vi "MakeReference.vi"(8 "error in (no error)":errorcluster, 10 "DatatoRef":T1, 11 "Refnum in":refnum<k34>) -> (0 "error out":errorcluster, 3 "Refnum out":refnum<k34>)   [LabVIEW 2021]
uses:
  Typedefs/DataToRef.ctl
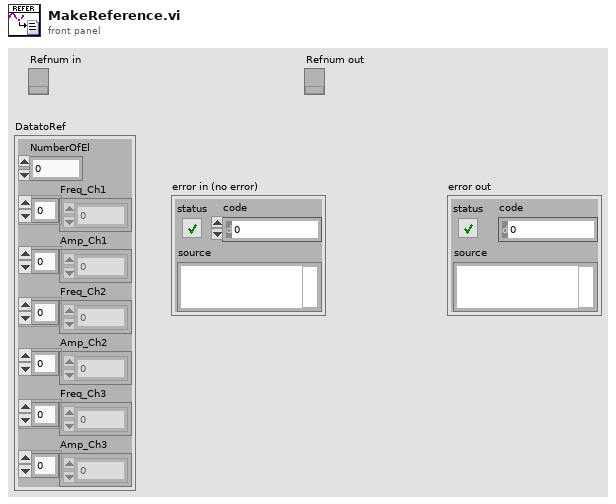
[diagram p1: front panel]
types:
  T1 = typedef "DataToRef.ctl" = cluster{"NumberOfEl":dbl, "Freq_Ch1":dbl[], "Amp_Ch1":dbl[], "Freq_Ch2":dbl[], "Amp_Ch2":dbl[], "Freq_Ch3":dbl[], "Amp_Ch3":dbl[]}
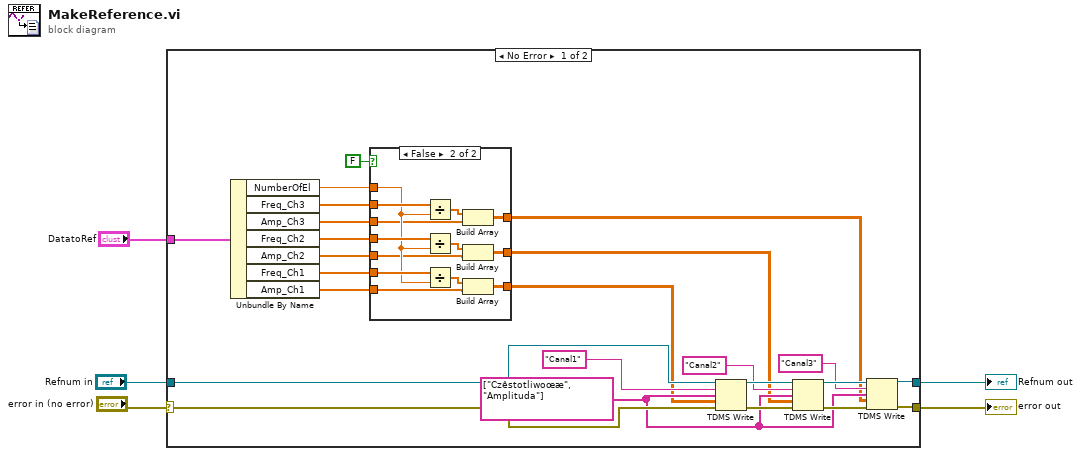
[diagram p0: block diagram]
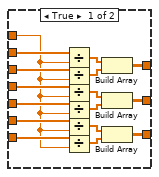
[diagram p2: hidden frame]
diagram:
  n1 = case shown="No Error" "error in (no error)" {
    selector: "error in (no error)" -> [w29 w59]
    tunnel: [w21 w59] -> w4
    tunnel: [w22 w60] -> w3
    tunnel: "Refnum in" -> [w28 w60]
    tunnel: "DatatoRef" -> [w17 _]
    frame No Error {
      w20 = string[] ["Czêstotliwoœæ", "Amplituda"] ("channel name(s) in (Untitled)")
      n2 = Unbundle By Name(w17) -> ("NumberOfEl"=w10:dbl, "Freq_Ch3"=w16:dbl[], "Amp_Ch3"=w15:dbl[], "Freq_Ch2"=w14:dbl[], "Amp_Ch2"=w13:dbl[], "Freq_Ch1"=w12:dbl[], "Amp_Ch1"=w11:dbl[])
      n3 = case shown="False" FALSE {
        tunnel: w16 -> [w45 w58]
        tunnel: w15 -> [w44 w48]
        tunnel: w14 -> [w43 w57]
        tunnel: w13 -> [w42 w47]
        tunnel: w12 -> [w41 w56]
        tunnel: w11 -> [w40 w46]
        tunnel: w10 -> [w39 w55]
        tunnel: [w32 w51] -> w9
        tunnel: [w31 w50] -> w8
        tunnel: [w30 w49] -> w7
        frame True {
          n4 = Divide(x=w45, y=w39) -> (x/y=w38:dbl[])
          n5 = Divide(x=w44, y=w39) -> (x/y=w37:dbl[])
          n6 = Divide(x=w43, y=w39) -> (x/y=w36:dbl[])
          n7 = Divide(x=w42, y=w39) -> (x/y=w35:dbl[])
          n8 = Divide(x=w41, y=w39) -> (x/y=w34:dbl[])
          n9 = Divide(x=w40, y=w39) -> (x/y=w33:dbl[])
          n10 = Build Array(w38, w37) -> (w32:dbl[][])
          n11 = Build Array(w36, w35) -> (w31:dbl[][])
          n12 = Build Array(w34, w33) -> (w30:dbl[][])
        }
        frame False {
          n13 = Divide(x=w58, y=w55) -> (x/y=w54:dbl[])
          n14 = Divide(x=w57, y=w55) -> (x/y=w53:dbl[])
          n15 = Divide(x=w56, y=w55) -> (x/y=w52:dbl[])
          n16 = Build Array(w54, w48) -> (w51:dbl[][])
          n17 = Build Array(w53, w47) -> (w50:dbl[][])
          n18 = Build Array(w52, w46) -> (w49:dbl[][])
        }
      }
      n19 = TDMS Write(0:w28, 5:"Canal1" ("group name in (Untitled)"), 7:w20, 9:w7, 11:w29) -> (4:w26:refnum<k34>, 15:w25:errorcluster)  [unwired: 1 in, 2 out]
      n20 = TDMS Write(0:w26, 5:"Canal2" ("group name in (Untitled)"), 7:w20, 9:w8, 11:w25) -> (4:w24:refnum<k34>, 15:w23:errorcluster)  [unwired: 1 in, 2 out]
      n21 = TDMS Write(0:w24, 5:"Canal3" ("group name in (Untitled)"), 7:w20, 9:w9, 11:w23) -> (4:w22:refnum<k34>, 15:w21:errorcluster)  [unwired: 1 in, 2 out]
    }
    frame Error {
    }
  }
  "error out" <- w4
  "Refnum out" <- w3
